vi "Streaming to Run Example.vi"() -> ()   [LabVIEW 2024]
doc: "Streams multiple channels to a Run."
uses:
  Sift API/Sift Client.lvclass
  Sift API/Types/Data Type.ctl
  Sift Client.lvlib
panel:
  out "Running":bool
  out "Run URL":string
  out "Flush Error":errorcluster
  in  "Test Channel 2":dbl(slide) scale=0.0..10.0
  in  "Stop":bool
  in  "Test Channel 1":dbl(slide) scale=0.0..10.0
  in  "Test Channel 3":bool
  in  "Run Name":string
  out "Error":errorcluster
  in  "Organization ID":string
  in  "API Key":string
  in  "API URL":string
  # "Sift Streaming Example"
  # "Instructions\n\n1. Fill in the API URL, API Key, and Organization ID. Visit this URL for more information on authentication\n    https://docs.siftstack.com/docs/api/authentication\n\n    Fill in a a name for the Run.\n\n2. Start the VI\n\n3. Navigate to the Run URL after it's populated to view the new Run.\n\n4. You should see the Sift Proxy and LabVIEW-Example in this Run.\n\n5. Click on the Live button and manually adjust the Controls to see the telemetry update.\n\n6. Click Stop to stop the VI."
  # "This example streams data live from LabVIEW.\n\nFill in the information below then open the corresponding Run in Sift\nto see data streaming in Live.\n\nNote: Remembver to hit the \"Live\" button after opening the run."
  # "(Open this link to view the Sift Run)"
  # "Adjust these values while streaming"
  # "Hit this to stop the example."
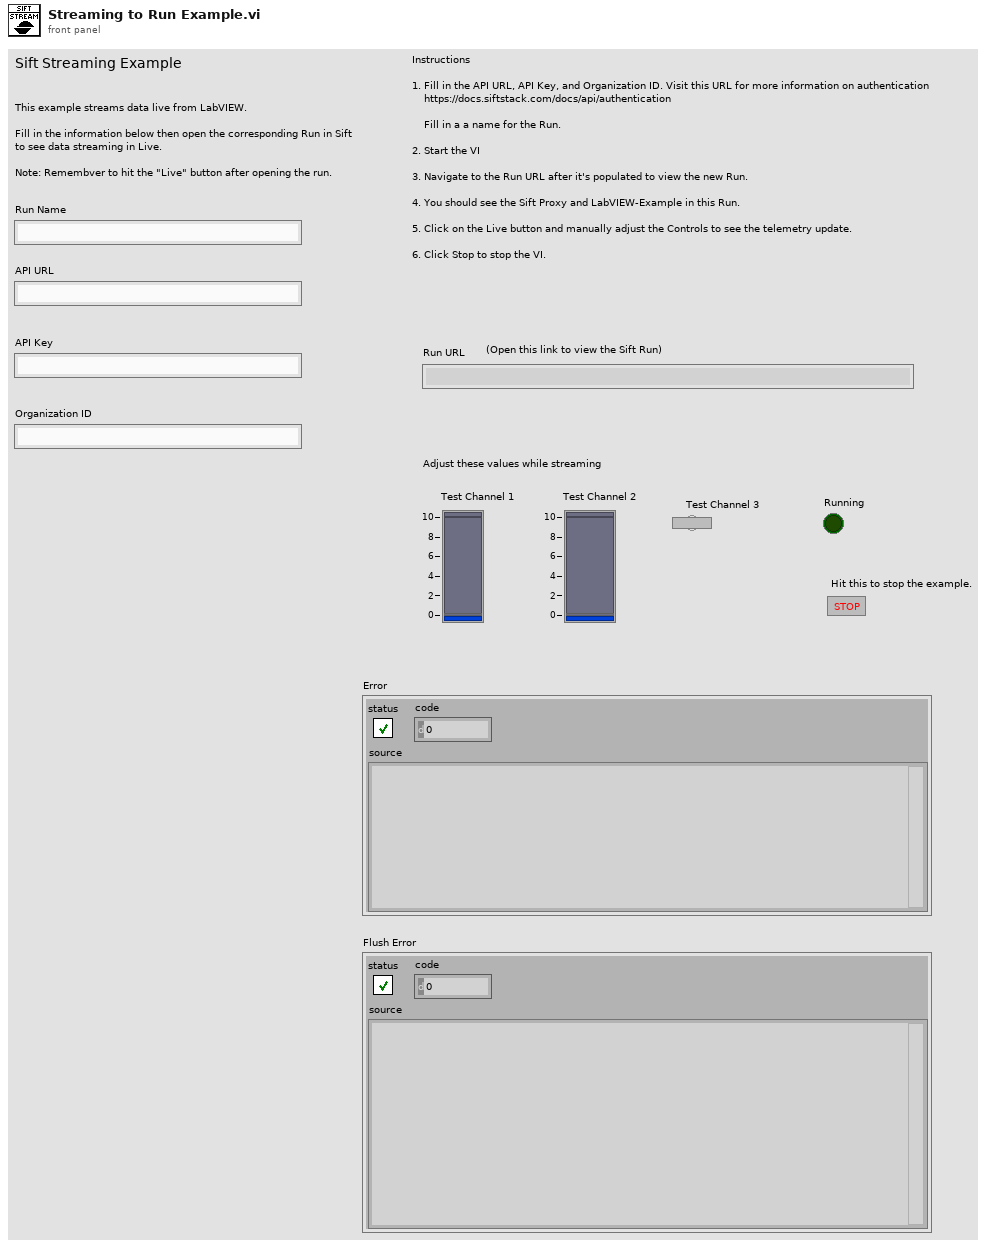
[diagram p1: front panel]
types:
  T1 = typedef "Sift Client.lvlib/Data Type.ctl" = enum8{"double", "float", "uint64", "int64", "uint32", "int32", "bool", "bit field", "enum"}
  T2 = typedef "Sift Client.lvlib/Timestamp.ctl" = cluster{"seconds":i64, "nanos":i32}
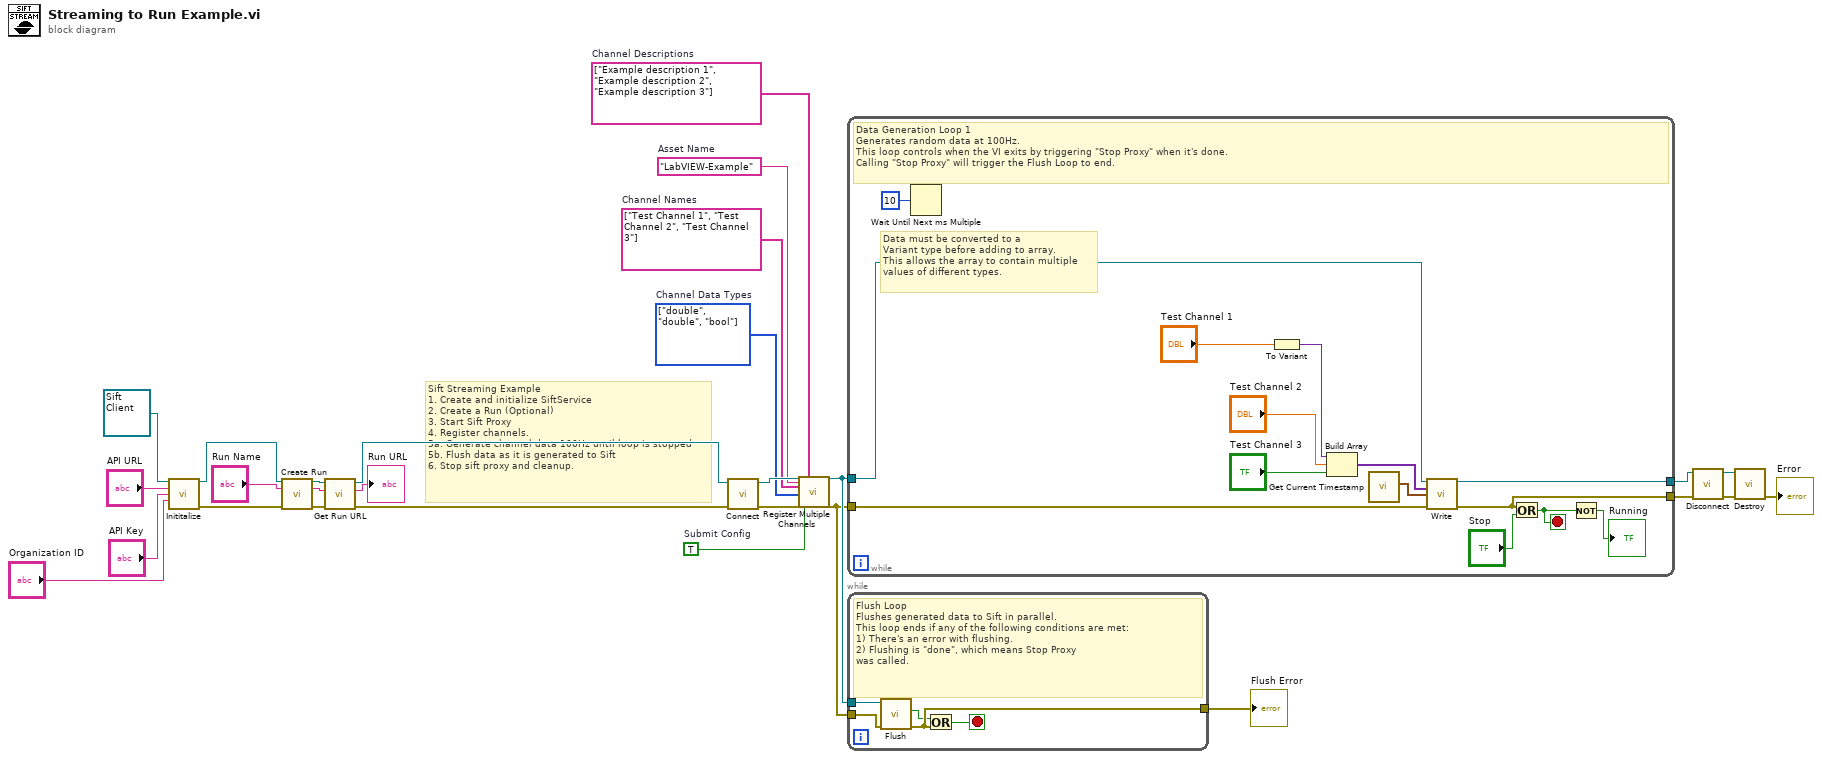
[diagram p0: block diagram]
diagram:
  w1 = TRUE  # Submit Config
  w13 = "LabVIEW-Example"  # Asset Name
  w15 = T1[] [enum."double", enum."double", enum."bool"] items=["double", "float", "uint64", "int64", "uint32", "int32", "bool", "bit field", "enum"]  # Channel Data Types
  w14 = string[] ["Example description 1", "Example description 2", "Example description 3"]  # Channel Descriptions
  w16 = string[] ["Test Channel 1", "Test Channel 2", "Test Channel 3"]  # Channel Names
  # "Sift Streaming Example\n1. Create and initialize SiftService\n2. Create a Run (Optional)\n3. Start Sift Proxy\n4. Register channels.\n5a. Generate channel data 100Hz until loop is stopped\n5b. Flush data as it is generated to Sift\n6. Stop sift proxy and cleanup."
  n1 = call-dynamic "Inititalize.vi"("Sift Client in"=refnum<class "Sift Client.lvclass"> refnum ("Sift Client.lvlib:Sift Client.lvclass"), "API URL"="API URL", "API Key"="API Key", "Organization ID"="Organization ID") -> ("Sift Client out"=w24:refnum<class "Sift Client.lvclass">, "error out"=w23:errorcluster)  [unwired: 10 in]
  n2 = call-dynamic "Create Run.vi"("Sift Client in"=w24, "Name"="Run Name", "error in (no error)"=w23) -> ("Sift Client out"=w3:refnum<class "Sift Client.lvclass">, "Run ID"=w7:string, "error out"=w5:errorcluster)  [unwired: 10 in]
  n3 = call-dynamic "Get Run URL.vi"("error in (no error)"=w5, "Run ID"=w7, "Sift Client in"=w3) -> ("error out"=w4:errorcluster, "URL"=→"Run URL":string, "Sift Client out"=w2:refnum<class "Sift Client.lvclass">)  [unwired: 6 in]
  n4 = call-dynamic "Connect.vi"("error in (no error)"=w4, "Sift Client in"=w2) -> ("error out"=w18:errorcluster, "Sift Client out"=w17:refnum<class "Sift Client.lvclass">)  [unwired: 7 in, 1 out]
  n5 = call "Register Multiple Channels.vi"("Sift Client in"=w17, "Asset Name"=w13, "Names"=w16, "Data Types"=w15, "error in (no error)"=w18, "Submit Config"=w1, "Descriptions"=w14) -> ("Sift Client out"=w10:refnum<class "Sift Client.lvclass">, "error out"=w8:errorcluster)  [unwired: 19 in]
  n6 = while {
    tunnel: w10 -> [w42]
    tunnel: w8 -> [w41]
    tunnel: [w34] -> w12
    tunnel: [w36] -> w11
    stop <- w29 stop-if-true
    # "Data must be converted to a \nVariant type before adding to array.\nThis allows the array to contain multiple \nvalues of different types."
    # "Data Generation Loop 1\nGenerates random data at 100Hz.\nThis loop controls when the VI exits by triggering \"Stop Proxy\" when it's done. \nCalling \"Stop Proxy\" will trigger the Flush Loop to end."
    n7 = Wait Until Next ms Multiple(millisecond multiple=u32 10 ("milliseconds to wait")) -> ()  [unwired: 1 out]
    n8 = To Variant(anything="Test Channel 1") -> (Variant=w39:variant)
    n9 = Build Array(w39, "Test Channel 2", "Test Channel 3") -> (w38:variant[])
    n10 = call "Get Current Timestamp.vi"() -> ("Timestamp"=w37:T2)  [unwired: 11 in]
    n11 = call-dynamic "Write.vi"("Sift Client in"=w42, "Values"=w38, "Timestamp"=w37, "error in (no error)"=w41) -> ("Sift Client out"=w34:refnum<class "Sift Client.lvclass">, "error out"=w36:errorcluster)  [unwired: 10 in]
    n12 = Or(x=w36, y="Stop") -> (x .or. y?=w29:bool)
    n13 = Not(x=w29) -> (.not. x?=→"Running":bool)
  }
  n14 = while {
    tunnel: w10 -> [w47]
    tunnel: [w45] -> w9
    tunnel: w8 -> [w46]
    stop <- w43 stop-if-true
    # "Flush Loop\nFlushes generated data to Sift in parallel.\nThis loop ends if any of the following conditions are met:\n1) There's an error with flushing.\n2) Flushing is \"done\", which means Stop Proxy \nwas called."
    n15 = call-dynamic "Flush.vi"("error in (no error)"=w46, "Sift Client in"=w47) -> ("error out"=w45:errorcluster, "Done"=w44:bool)  [unwired: 7 in, 1 out]
    n16 = Or(x=w44, y=w45) -> (x .or. y?=w43:bool)
  }
  "Flush Error" <- w9
  n17 = call-dynamic "Disconnect.vi"("error in (no error)"=w11, "Sift Client in"=w12) -> ("error out"=w21:errorcluster, "Sift Client out"=w20:refnum<class "Sift Client.lvclass">)  [unwired: 8 in]
  n18 = call-dynamic "Destroy.vi"("error in (no error)"=w21, "Sift Client in"=w20) -> ("error out"=→"Error":errorcluster)  [unwired: 8 in, 1 out]
